vi "Velox_ReadChuckStatus.vi"(8 "error in (no error)":errorcluster, 11 "VeloxTeslaProbestation in":refnum<class "VeloxTeslaProbestation.lvclass">) -> (0 "error out":errorcluster, 2 "Status":T1, 3 "VeloxTeslaProbestation out":refnum<class "VeloxTeslaProbestation.lvclass">)   [LabVIEW 2018, in "VeloxTeslaProbestation.lvclass"]
uses:
  VeloxTeslaProbestation.lvclass
  Desktop/Kvasnicka/test_labview_library/Integration_toolkit_library/CascadeProbestation.lvlib
panel:
  out "Response":string
  out "Chuck camera":T2(ring)
  out "lift up?":bool
  out "Load position":T3
  out "Z Height":T4(ring)
  out "Compensation mode":enum8{"None", "Prober", "Offset", "Technology"}(ring)
  out "Vacuum on?":bool
  out "IsMoving":T5
  out "OnEndLimit":T6
  out "Mode":T7
  out "IsInitialized":T8
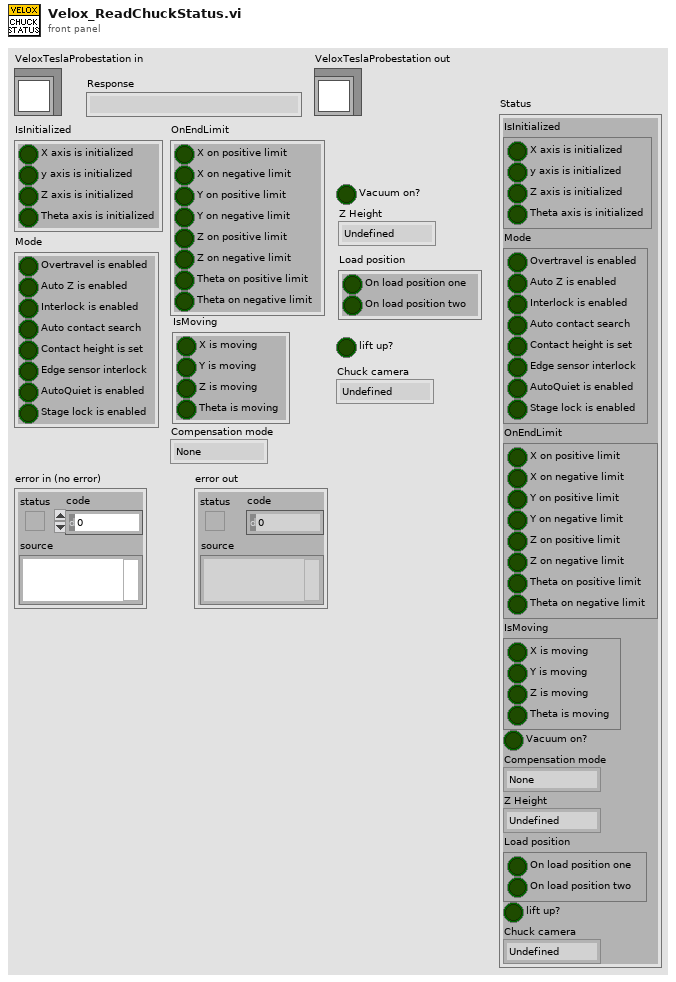
[diagram p1: front panel]
types:
  T1 = cluster{"IsInitialized":cluster{"X axis is initialized":bool, "y axis is initialized":bool, "Z axis is initialized":bool, "Theta axis is initialized":bool}, "Mode":cluster{"Overtravel is enabled":bool, "Auto Z is enabled":bool, "Interlock is enabled":bool, "Auto contact search":bool, "Contact height is set":bool, "Edge sensor interlock":bool, "AutoQuiet is enabled":bool, "Stage lock is enabled":bool}, "OnEndLimit":cluster{"X on positive limit":bool, "X on negative limit":bool, "Y on positive limit":bool, "Y on negative limit":bool, "Z on positive limit":bool, "Z on negative limit":bool, "Theta on positive limit":bool, "Theta on negative limit":bool}, "IsMoving":cluster{"X is moving":bool, "Y is moving":bool, "Z is moving":bool, "Theta is moving":bool}, "Vacuum on?":bool, "Compensation mode":enum8{"None", "Prober", "Offset", "Technology"}, "Z Height":enum8{"Undefined", "Search", "Overtravel", "Alignment", "Separation", "Contact"}, "Load position":cluster{"On load position one":bool, "On load position two":bool}, "lift up?":bool, "Chuck camera":enum8{"Undefined", "On chuck", "At park position"}}
  T2 = enum8{"Undefined", "On chuck", "At park position"}
  T3 = cluster{"On load position one":bool, "On load position two":bool}
  T4 = enum8{"Undefined", "Search", "Overtravel", "Alignment", "Separation", "Contact"}
  T5 = cluster{"X is moving":bool, "Y is moving":bool, "Z is moving":bool, "Theta is moving":bool}
  T6 = cluster{"X on positive limit":bool, "X on negative limit":bool, "Y on positive limit":bool, "Y on negative limit":bool, "Z on positive limit":bool, "Z on negative limit":bool, "Theta on positive limit":bool, "Theta on negative limit":bool}
  T7 = cluster{"Overtravel is enabled":bool, "Auto Z is enabled":bool, "Interlock is enabled":bool, "Auto contact search":bool, "Contact height is set":bool, "Edge sensor interlock":bool, "AutoQuiet is enabled":bool, "Stage lock is enabled":bool}
  T8 = cluster{"X axis is initialized":bool, "y axis is initialized":bool, "Z axis is initialized":bool, "Theta axis is initialized":bool}
  T9 = cluster{"Boolean array[0]":bool, "Boolean array[1]":bool, "Boolean array[2]":bool, "Boolean array[3]":bool}
  T10 = cluster{"Boolean array[0]":bool, "Boolean array[1]":bool}
  T11 = cluster{"Boolean array[0]":bool, "Boolean array[1]":bool, "Boolean array[2]":bool, "Boolean array[3]":bool, "Boolean array[4]":bool, "Boolean array[5]":bool, "Boolean array[6]":bool, "Boolean array[7]":bool}
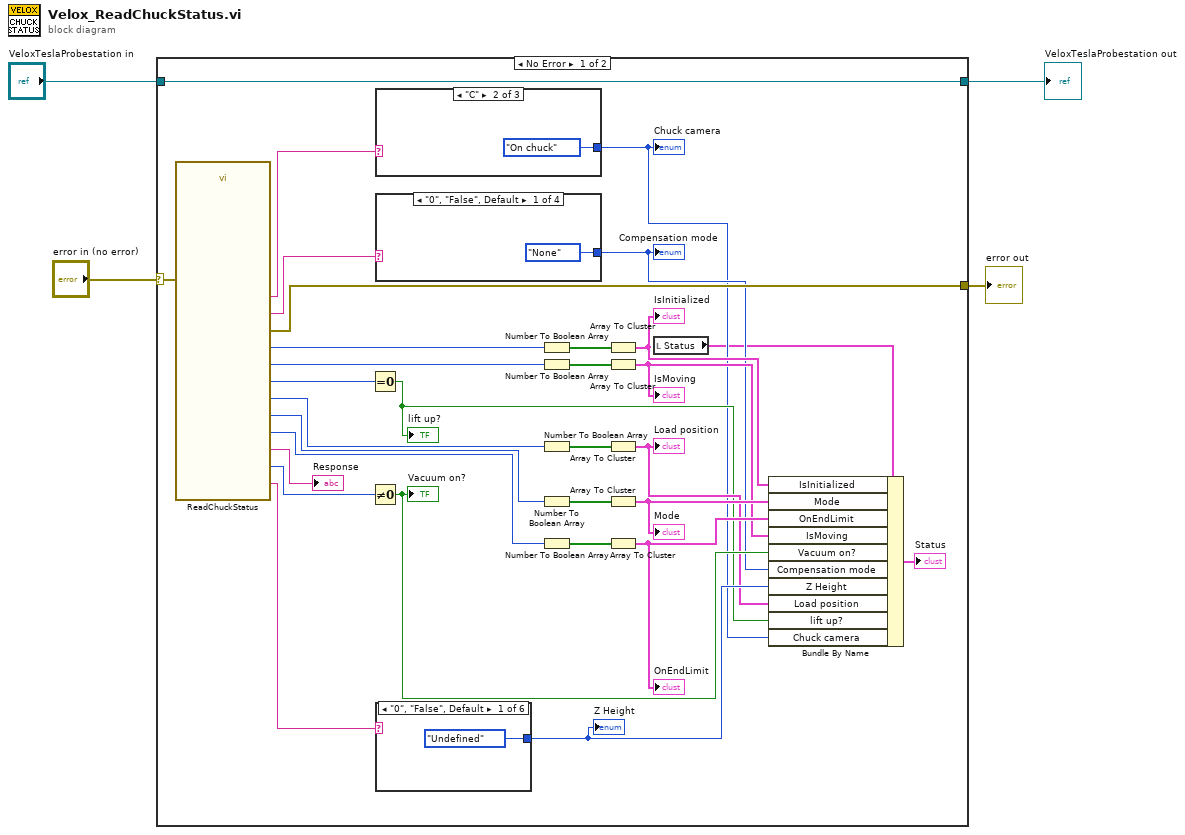
[diagram p0: block diagram]
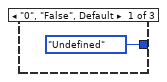
[diagram p2: hidden frame]
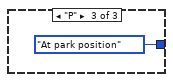
[diagram p3: hidden frame]
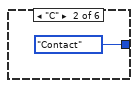
[diagram p4: hidden frame]
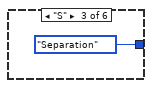
[diagram p5: hidden frame]
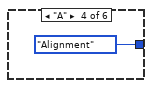
[diagram p6: hidden frame]
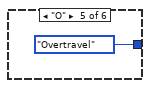
[diagram p7: hidden frame]
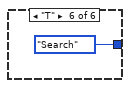
[diagram p8: hidden frame]
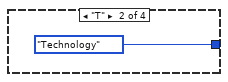
[diagram p9: hidden frame]
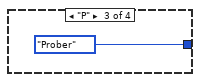
[diagram p10: hidden frame]
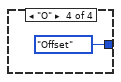
[diagram p11: hidden frame]
diagram:
  n1 = case shown="No Error" "error in (no error)" {
    selector: "error in (no error)" -> [w34 w50]
    tunnel: [w33 w50] -> w3
    tunnel: [w35 w49] -> w1
    tunnel: "VeloxTeslaProbestation in" -> [w35 w49]
    frame No Error {
      n2 = call "ReadChuckStatus.vi"("Error In"=w34) -> ("ChuckCamera"=w18:string, "Vacuum"=w24:i32, "Z Height"=w22:string, "Load Pos"=w19:i32, "CompMode"=w23:string, "Lift"=w21:i32, "Response"=→"Response":string, "IsInitialized"=w32:i32, "Mode"=w30:i32, "OnEndLimit"=w27:i32, "IsMoving"=w25:i32, "Error Out"=w33:errorcluster)  [unwired: 7 in]
      n3 = Equal To 0?(x=w21) -> (x = 0?=w9:bool)
      "lift up?" <- w9
      n4 = Not Equal To 0?(x=w24) -> (x != 0?=w13:bool)
      "Vacuum on?" <- w13
      n5 = case shown="\"C\"" w18 {
        tunnel: [T2."Undefined" ("Chuck camera") T2."On chuck" ("Chuck camera") T2."At park position" ("Chuck camera")] -> w8
        frame "0", "False", Default {
        }
        frame "C" {
        }
        frame "P" {
        }
      }
      "Chuck camera" <- w8
      n6 = case shown="\"0\", \"False\", Default" w23 {
        tunnel: [enum8{"None", "Prober", "Offset", "Technology"}."None" ("Enum") enum8{"None", "Prober", "Offset", "Technology"}."Technology" ("Enum") enum8{"None", "Prober", "Offset", "Technology"}."Prober" ("Enum") enum8{"None", "Prober", "Offset", "Technology"}."Offset" ("Enum")] -> w12
        frame "0", "False", Default {
        }
        frame "T" {
        }
        frame "P" {
        }
        frame "O" {
        }
      }
      "Compensation mode" <- w12
      n7 = case shown="\"0\", \"False\", Default" w22 {
        tunnel: [T4."Undefined" ("Z Height") T4."Contact" ("Z Height") T4."Separation" ("Z Height") T4."Alignment" ("Z Height") T4."Overtravel" ("Z Height") T4."Search" ("Z Height")] -> w11
        frame "0", "False", Default {
        }
        frame "C" {
        }
        frame "S" {
        }
        frame "A" {
        }
        frame "O" {
        }
        frame "T" {
        }
      }
      "Z Height" <- w11
      n8 = Number To Boolean Array(number=w32) -> (Boolean array=w31:bool[])
      n9 = Number To Boolean Array(number=w25) -> (Boolean array=w26:bool[])
      n10 = Number To Boolean Array(number=w19) -> (Boolean array=w20:bool[])
      n11 = Number To Boolean Array(number=w30) -> (Boolean array=w29:bool[])
      n12 = Number To Boolean Array(number=w27) -> (Boolean array=w28:bool[])
      n13 = Array To Cluster(array=w31) -> (cluster=w17:T9)
      "IsInitialized" <- w17
      n14 = Array To Cluster(array=w26) -> (cluster=w14:T9)
      "IsMoving" <- w14
      n15 = Array To Cluster(array=w20) -> (cluster=w10:T10)
      "Load position" <- w10
      n16 = Array To Cluster(array=w29) -> (cluster=w16:T11)
      "Mode" <- w16
      n17 = Array To Cluster(array=w28) -> (cluster=w15:T11)
      "OnEndLimit" <- w15
      n18 = local read "Status"() -> (w6:T1)
      n19 = Bundle By Name(cluster=w6, "IsInitialized"=w17, "Mode"=w16, "OnEndLimit"=w15, "IsMoving"=w14, "Vacuum on?"=w13, "Compensation mode"=w12, "Z Height"=w11, "Load position"=w10, "lift up?"=w9, "Chuck camera"=w8) -> (→"Status":T1)
    }
    frame Error {
    }
  }
  "error out" <- w3
  "VeloxTeslaProbestation out" <- w1
